vi "TracePoint.vi"() -> (3 "template trace point":string)   [LabVIEW 2017, in "EmsaDataFlowManager.lvlib"]
uses:
  <vilib>/addons/InsightCM/Devices/Shared/Emsa/EmsaDataFlowManager/EmsaDataFlowManager.lvlib
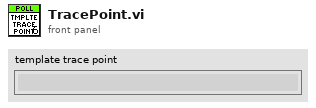
[diagram p1: front panel]
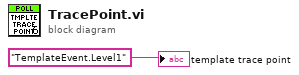
[diagram p0: block diagram]
diagram:
  "template trace point" <- "TemplateEvent.Level1" ("ProcessName")
